vi "AWS-S3-ClientRef-Set.vi"(8 "S3 Client ref":refnum<k24>, 11 "AWS-S3-API":refnum<class "AWS-S3-API.lvclass">) -> (3 "AWS-S3-API out":refnum<class "AWS-S3-API.lvclass">)   [LabVIEW 2012, in "AWS-S3-API.lvclass"]
uses:
  AWS-S3-API.lvclass
  C:/Users/Jack/repo/aws/AWS-SDK/AWSSDK.dll
  repo/aws/AWS-SDK/AWSSDK.dll
panel:
  # "Inputs"
  # "Outputs"
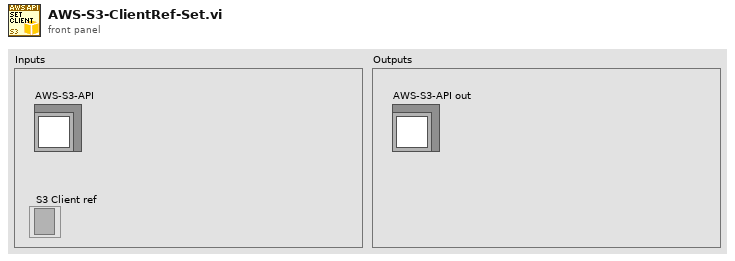
[diagram p1: front panel]
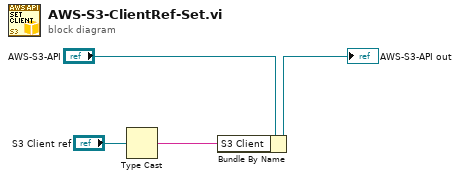
[diagram p0: block diagram]
diagram:
  n1 = Type Cast(x="S3 Client ref") -> (*(type *) &x=w1:string)  [unwired: 1 in]
  n2 = Bundle By Name(cluster="AWS-S3-API", "S3 Client"=w1) -> (→"AWS-S3-API out":refnum<class "AWS-S3-API.lvclass">)
